vi "Return_All_Scopes.vi"(9 "Password":string, 10 "User Name":string, 11 "Target (localhost)":refnum<k21>="localhost") -> (2 "Array":T1[](array[typedef]))   [LabVIEW 2021]
doc: "Displays all hardware and certain properties of that hardware on the specified target."
uses:
  C:/Users/NI/Desktop/SCPI_Scope/Controls/Clusts/Scope_Details_Clust.ctl
  <vilib>/nisyscfg/Filter Mode.ctl
  786f16a0-9eb0-424a-b110-95e7cb814a15.vi
  <vilib>/Array/Sort 2D Array - Pop Stack.vi
  <vilib>/Array/Sort 2D Array - Push Stack.vi
  <vilib>/nisyscfg/Close (Hardware).vi
  <vilib>/nisyscfg/Close (Filter).vi
  <vilib>/nisyscfg/Close (System).vi
  <instrlib>/niScope/Utility/niScope Get Channel Name.vi
  <vilib>/nisyscfg/nisyscfg.lvlib
  <resource>/objmgr/nicontrollersysapi.rc
  <resource>/objmgr/niflexrioatomicsae.rc
panel:
  out "error out":errorcluster
  out "LoopCount":i32
  out "Resources":string[][](table)
  # "Overview: Displays all hardware and certain properties of that hardware on the specified target.\nRequirements: NI System Configuration, applicable device drivers\nInstructions:\n1. Select Target. Enter User Name and Password if necessary.\n2. Run the VI."
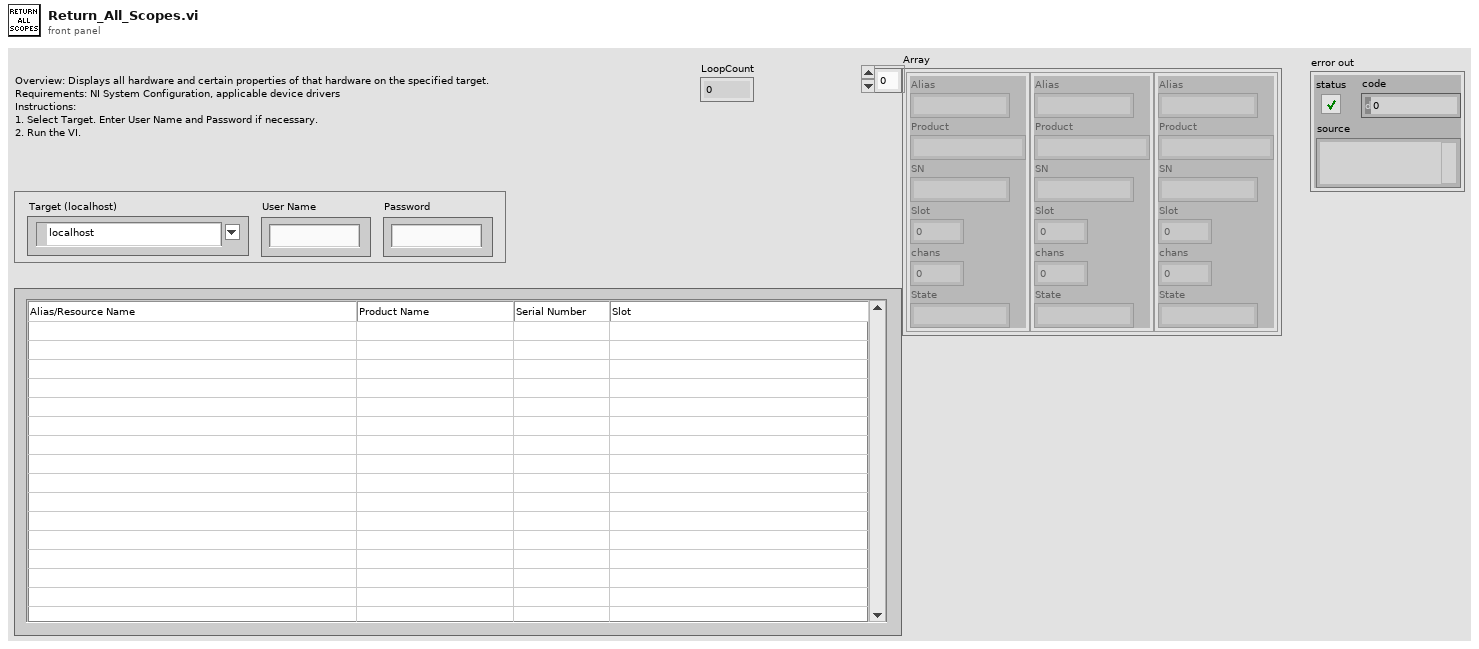
[diagram p1: front panel]
types:
  T1 = typedef "Scope_Details_Clust.ctl" = cluster{"Alias":string, "Product":string, "SN":string, "Slot":i32, "chans":i32, "State":string}
  T2 = typedef "nisyscfg.lvlib/Filter Mode.ctl" = i32
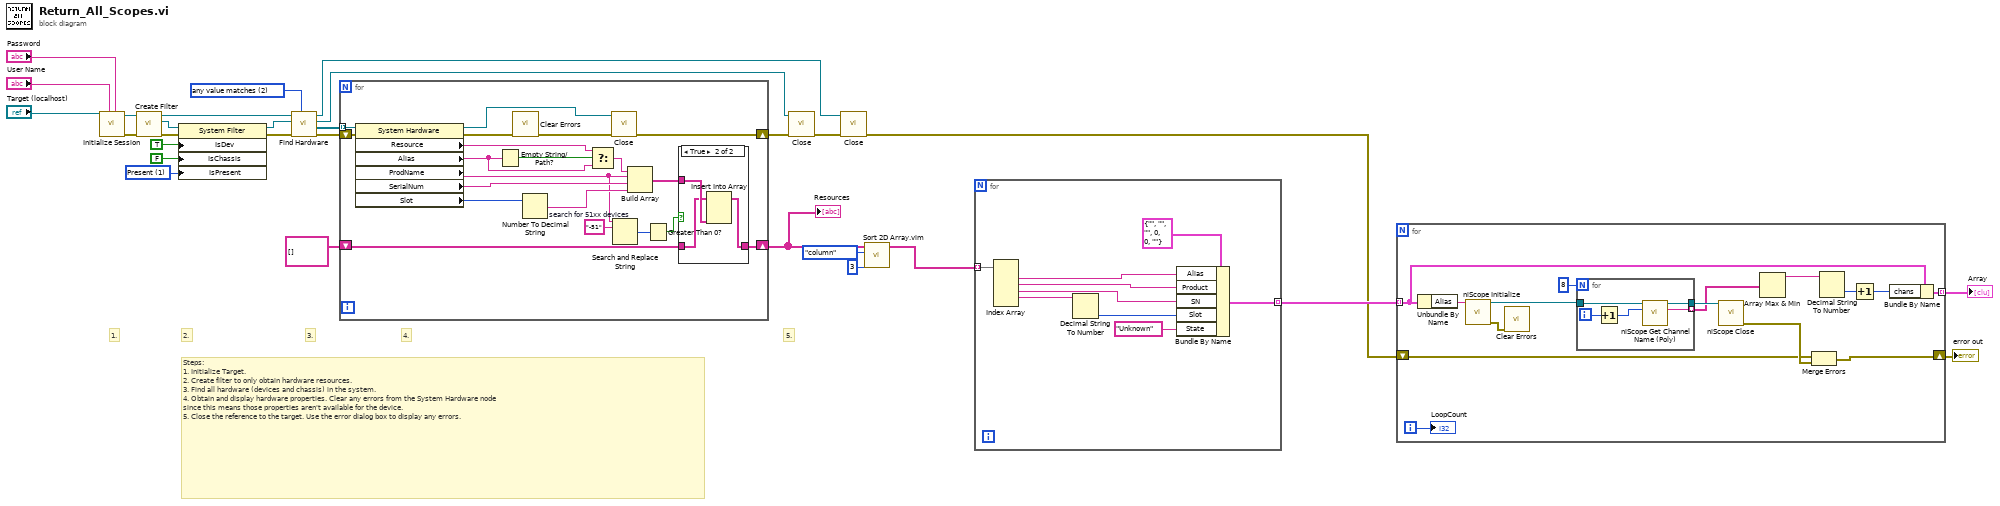
[diagram p0: block diagram]
diagram:
  w10 = 1 items=["Initializing"=-2, "Unknown"=-1, "Not Present"=0, "Present"=1] ("Devices & Chassis:Is Present")
  w19 = T2 2 items=["all values match"=1, "any value matches"=2, "values do not match"=3, "all properties exist"=4] ("filter mode (all values match)")
  # "2."
  # "5."
  # "4."
  # "3."
  # "1."
  # "Steps:\n1. Initialize Target.\n2. Create filter to only obtain hardware resources.\n3. Find all hardware (devices and chassis) in the system.\n4. Obtain and display hardware properties. Clear any errors from the System Hardware node\nsince this means those properties aren't available for the device. \n5. Close the reference to the target. Use the error dialog box to display any errors."
  n1 = call <vilib>:"Initialize Session.vi"("Password"="Password", "User Name"="User Name", "Target (localhost)"="Target (localhost)") -> ("error out"=w21:errorcluster, "Session out"=w24:refnum<k21>)  [unwired: 7 in]
  n2 = call <vilib>:"Create Filter.vi"("error in (no error)"=w21, "Session in"=w24) -> ("error out"=w26:errorcluster, "Filter out"=w25:refnum<k20>, "Session out"=w23:refnum<k21>)  [unwired: 7 in]
  n3 = property class="System Filter"(reference=w25, error in=w26, "IsDev"=TRUE ("Is Chassis"), "IsChassis"=FALSE ("Is Chassis"), "IsPresent"=w10) -> (reference out=w20:refnum<k20>, error out=w22:errorcluster)
  n4 = call <vilib>:"Find Hardware.vi"("Filter Mode (all values match)"=w19, "error in (no error)"=w22, "Filter in"=w20, "Session in"=w23) -> ("error out"=w15:errorcluster, "Resources out"=w29:refnum<k20>[], "Filter out"=w17:refnum<k20>, "Session out"=w27:refnum<k21>)  [unwired: 4 out]
  n5 = for {
    tunnel: w29 -> [w47] mode=indexing
    shift-right: [w49] -> w16
    shift-left: w15 -> [w41]
    shift-right: [w40] -> w1
    shift-left: string[][] [] ("Results") -> [w38]
    w32 = "-51"  # search for 51xx devices
    n6 = property class="System Hardware"(reference=w47, error in=w41) -> (reference out=w42:refnum<k20>, error out=w43:errorcluster, "Resource"=w45:string, "Alias"=w46:string, "ProdName"=w33:string, "SerialNum"=w44:string, "Slot"=w35:i32)
    n7 = Empty String/Path?(string/path=w46) -> (empty?=w48:bool)
    n8 = call <vilib>:"Clear Errors.vi"("error in (no error)"=w43) -> ("error out"=w37:errorcluster)  [unwired: 5 in, 1 out]
    n9 = Number To Decimal String(number=w35) -> (decimal integer string=w34:string)  [unwired: 1 in]
    n10 = Select(t=w45, s=w48, f=w46) -> (s? t:f=w36:string)
    n11 = call-poly <vilib>:"Close.vi"("error in (no error)"=w37, "Resource in"=w42) -> ("error out"=w49:errorcluster)  [unwired: 9 in]
    n12 = Search and Replace String(input string=w33, search string=w32) -> (number of replacements=w31:i32)  [unwired: 6 in, 3 out]
    n13 = Build Array(w36, w33, w44, w34) -> (w39:string[])
    n14 = Greater Than 0?(x=w31) -> (x > 0?=w30:bool)
    n15 = case shown="True" w30 {
      tunnel: [w50 w53] -> w40
      tunnel: w39 -> [_ w52]
      tunnel: w38 -> [w50 w51]
      frame False {
      }
      frame True {
        n16 = Insert Into Array(array=w51, new element=w52) -> (w53:string[][])  [unwired: 2 in]
      }
    }
  }
  "Resources" <- w1
  n17 = call-poly <vilib>:"Close.vi"("error in (no error)"=w16, "Filter in"=w17) -> ("error out"=w18:errorcluster)  [unwired: 9 in]
  n18 = call-poly <vilib>:"Close.vi"("error in (no error)"=w18, "Session in"=w27) -> ("error out"=w4:errorcluster)  [unwired: 9 in]
  n19 = call "Sort 2D Array.vim"("index"=3, "dimension to index (column)"=enum16{"column", "row"}."column", "2D array"=w1) -> ("sorted 2D array"=w7:string[][])  [unwired: 7 in, 1 out]
  n20 = for {
    tunnel: w7 -> [w62] mode=indexing
    tunnel: [w54] -> w6 mode=indexing
    n21 = Index Array(array=w62) -> (element #1=w60:string, element #2=w59:string, element #3=w58:string, element #4=w57:string)  [unwired: 5 in, 1 out]
    n22 = Decimal String To Number(string=w57) -> (number=w55:i32)  [unwired: 2 in, 1 out]
    n23 = Bundle By Name(cluster=T1 {"Alias"="", "Product"="", "SN"="", "Slot"=0, "chans"=0, "State"=""} ("ScopeDetails"), "Alias"=w60, "Product"=w59, "SN"=w58, "Slot"=w55, "State"="Unknown") -> (w54:T1)
  }
  n24 = for {
    tunnel: w6 -> [w72] mode=indexing
    tunnel: [w71] -> w5 mode=indexing
    shift-right: [w63] -> w3
    shift-left: w4 -> [w64]
    i -> [w77]
    n25 = Unbundle By Name(w72) -> ("Alias"=w76:string)
    n26 = call <instrlib>:"niScope Initialize.vi"("resource name"=w76) -> ("instrument handle"=w75:refnum<k15>, "error out"=w66:errorcluster)  [unwired: 13 in]
    n27 = call <vilib>:"Clear Errors.vi"("error in (no error)"=w66) -> ()  [unwired: 5 in, 2 out]
    n28 = for {
      N: 8 -> [_]
      tunnel: [w82] -> w70 mode=indexing
      tunnel: w75 -> [w81]
      tunnel: [w80] -> w74
      i -> [w79]
      n29 = Increment(x=w79) -> (x+1=w78:i32)
      n30 = call-poly <instrlib>:"niScope Get Channel Name (Poly).vi"("instrument handle"=w81, "index"=w78) -> ("instrument handle out"=w80:refnum<k15>, "channel name"=w82:string)  [unwired: 11 in, 1 out]
    }
    n31 = call <instrlib>:"niScope Close.vi"("instrument handle"=w74) -> ("error out"=w65:errorcluster)  [unwired: 14 in]
    n32 = Array Max & Min(array=w70) -> (max value=w69:string)  [unwired: 3 out]
    n33 = Merge Errors(w64, w65) -> (w63:errorcluster)
    n34 = Decimal String To Number(string=w69) -> (number=w68:i32)  [unwired: 2 in, 1 out]
    n35 = Increment(x=w68) -> (x+1=w67:i32)
    n36 = Bundle By Name(cluster=w72, "chans"=w67) -> (w71:T1)
    "LoopCount" <- w77
  }
  "Array" <- w5
  "error out" <- w3
